vi "Skeleton extraction algorithm (zhangSuen algorithm).vi"() -> ()   [LabVIEW 2021]
panel:
  in  "Input array":dbl[][](array[numeric])=array290x480[139200 elements]
  out "自动迭代次数\nNumber of automatic iterations":i32=4
  in  "automatic 是否自动":bool=TRUE
  out "Step 2":dbl[][](graph)
  in  "指定Zhang-Suen\n     循环次数\nSpecify the number of Zhang-Suen cycles":i32
  out "x与y？":bool
  out "Step 1":dbl[][](graph)
  # "大津算法"
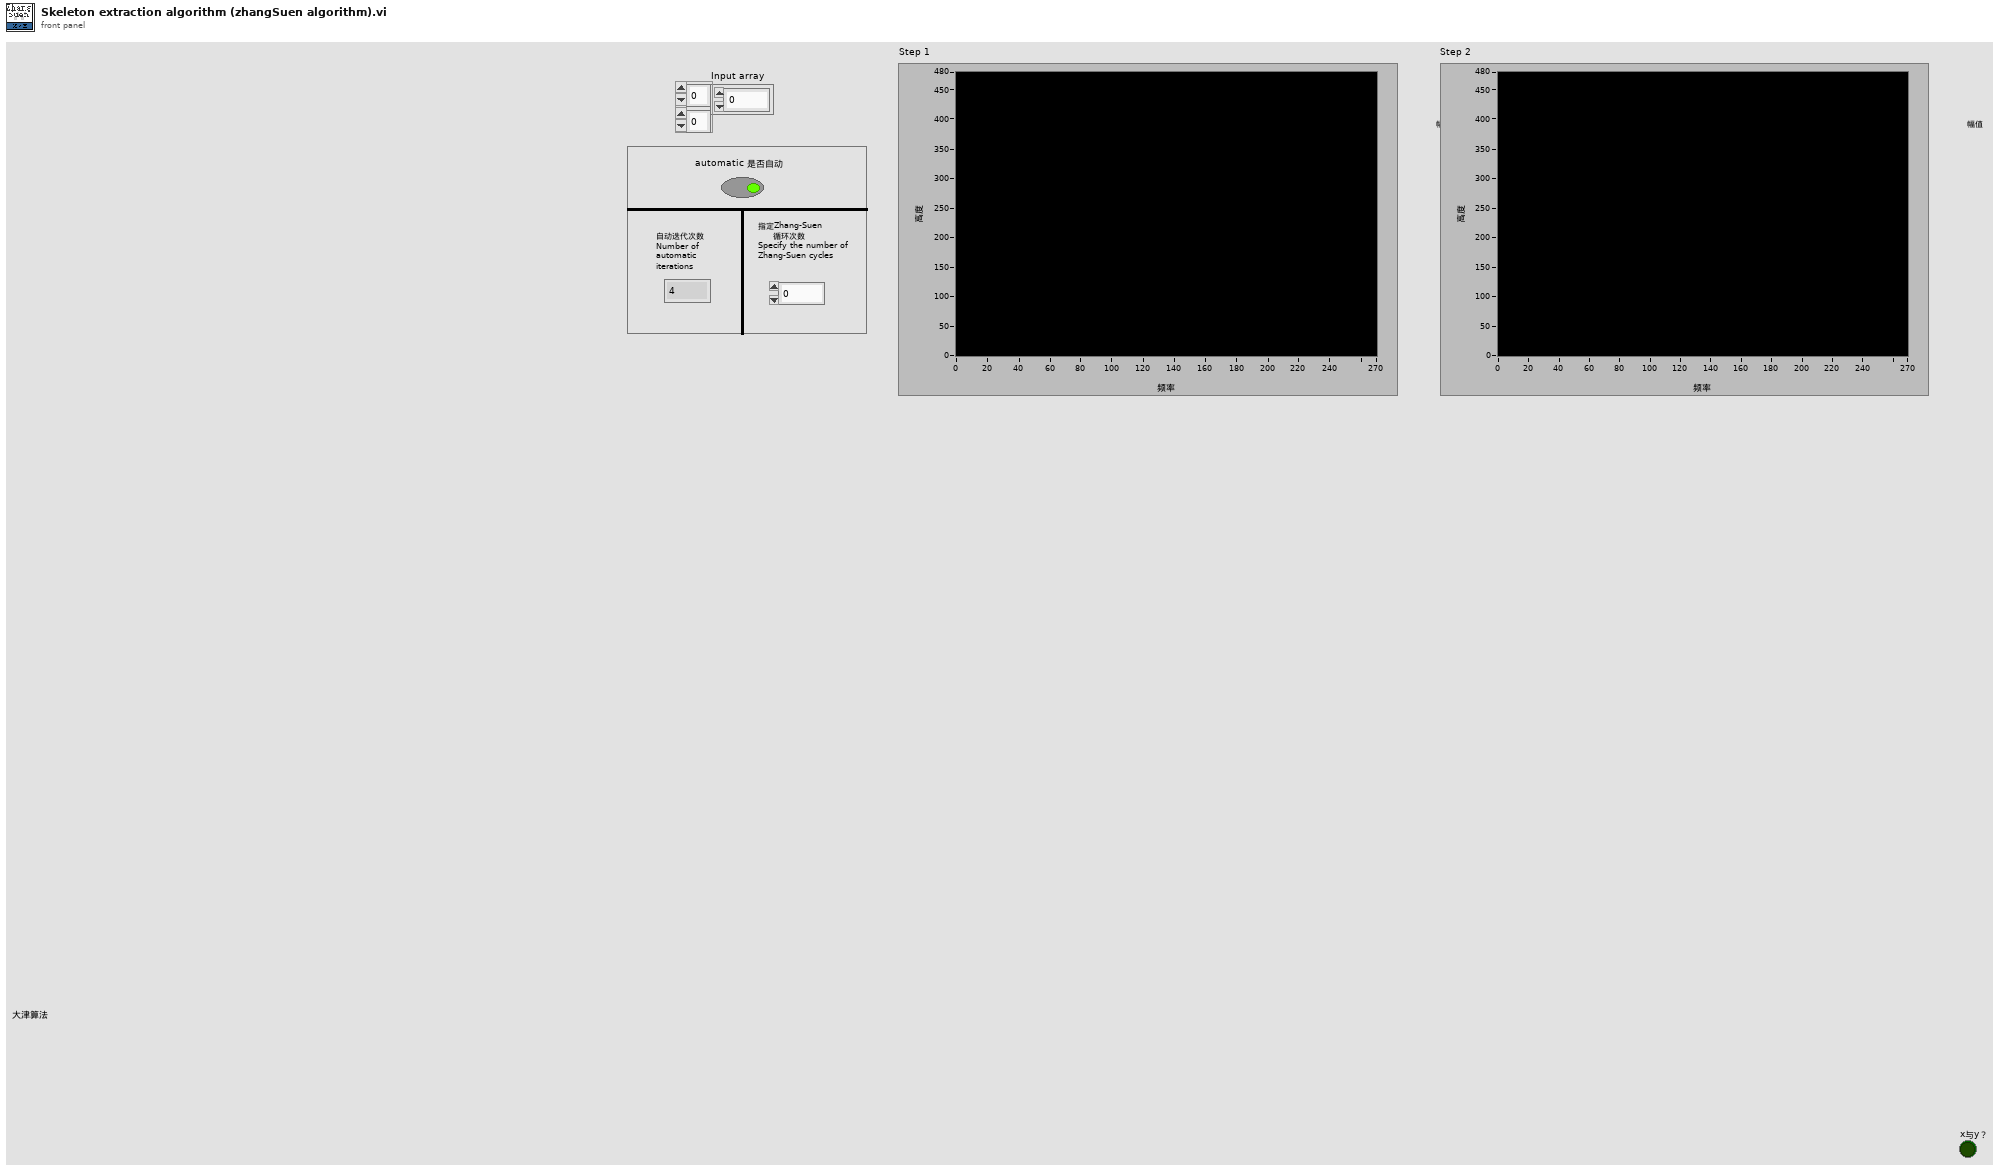
[diagram p1: front panel]
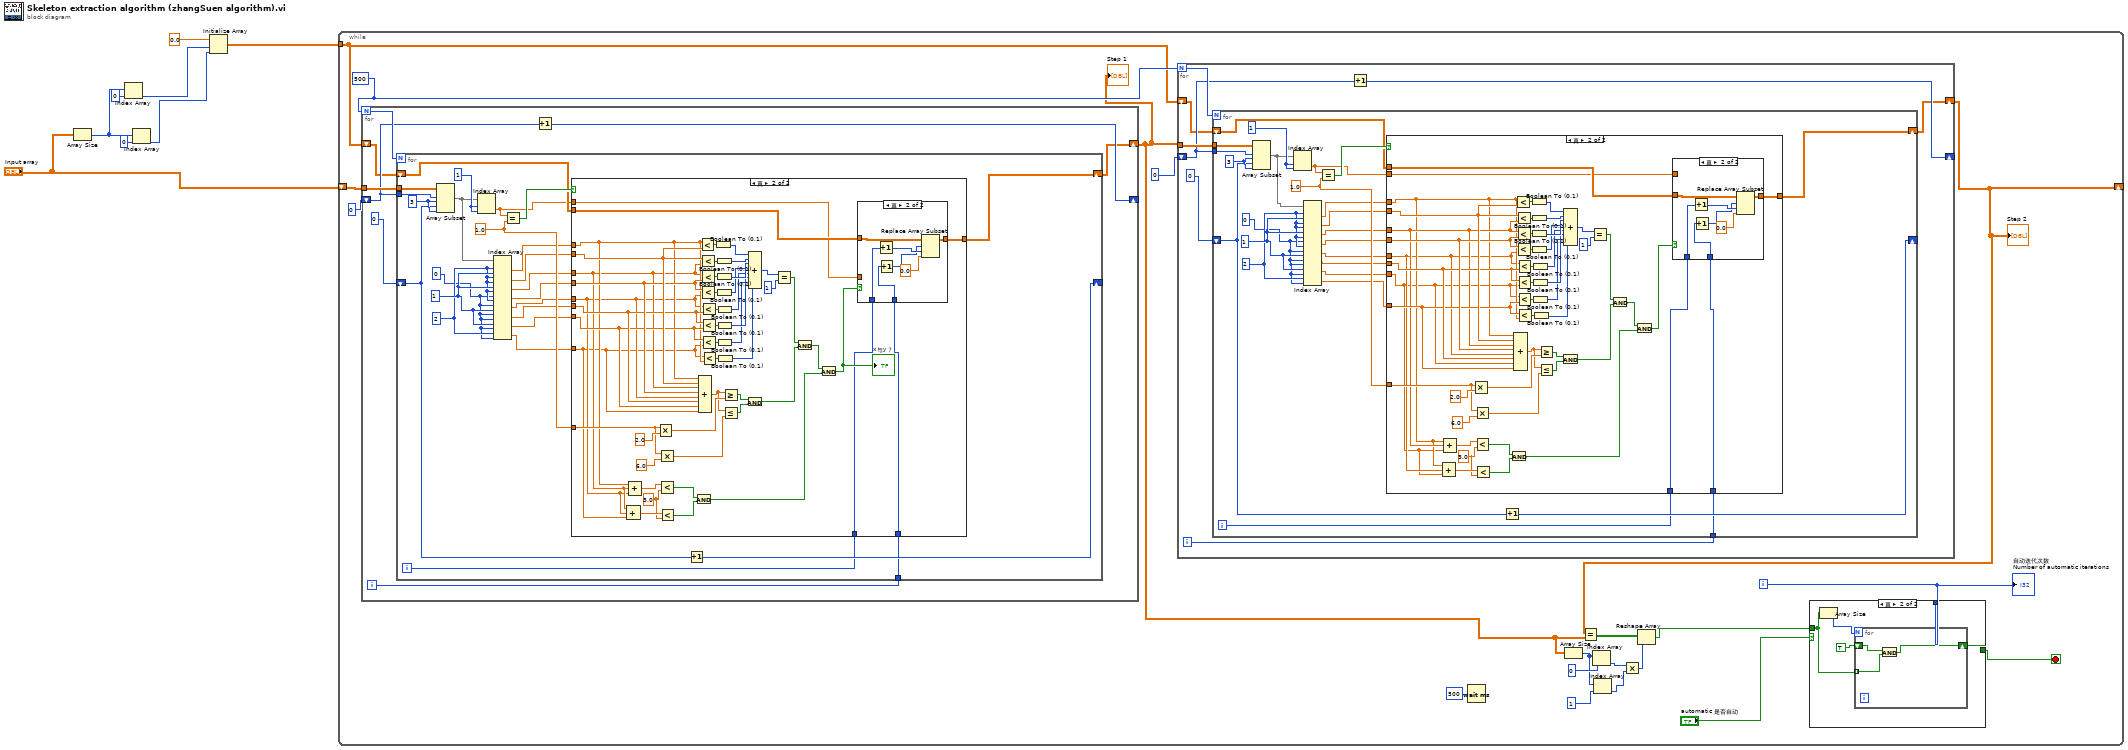
[diagram p0: block diagram]
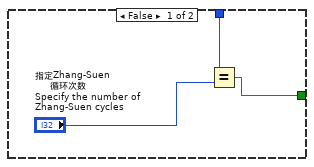
[diagram p2: hidden frame]
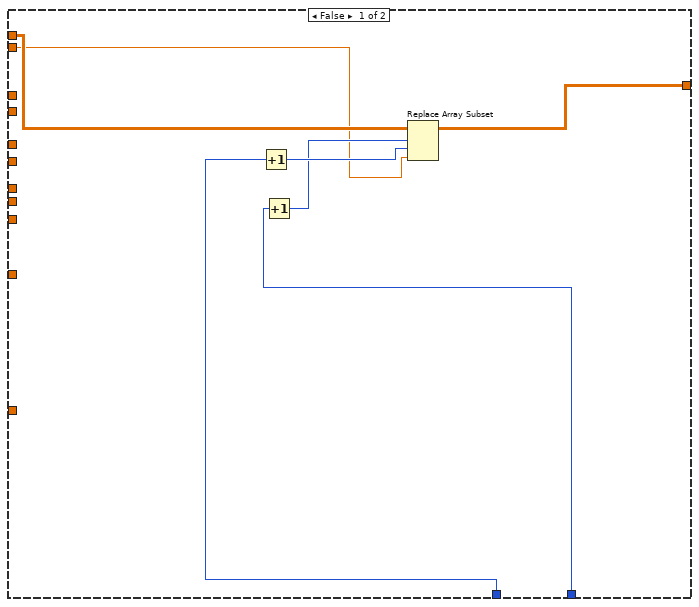
[diagram p3: hidden frame]
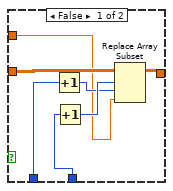
[diagram p4: hidden frame]
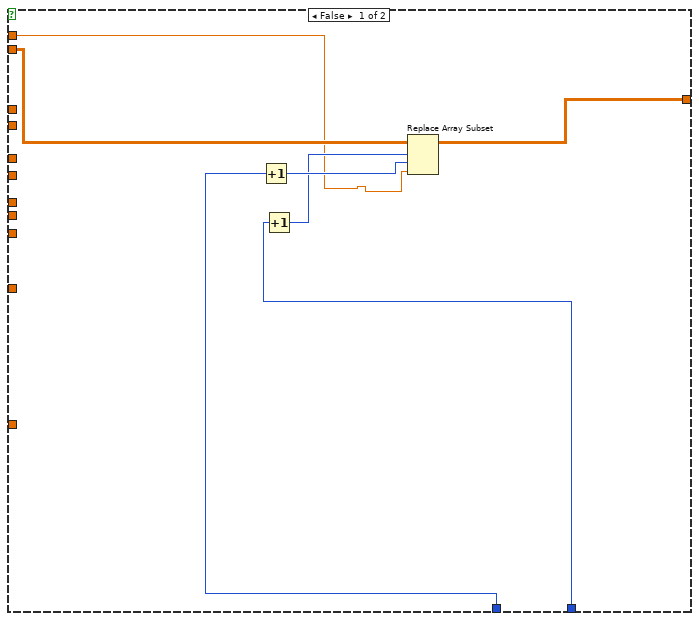
[diagram p5: hidden frame]
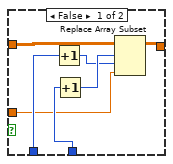
[diagram p6: hidden frame]
diagram:
  n1 = Array Size(array="Input array") -> (size(s)=w2:i32[])
  n2 = Index Array(array=w2, index=0 ("索引")) -> (element=w4:i32)
  n3 = Index Array(array=w2, index=0 ("索引")) -> (element=w1:i32)
  n4 = Initialize Array(0.0 ("元素"), w4, w1) -> (w7:dbl[][])
  n5 = while {
    tunnel: w7 -> [w24]
    shift-right: [w19] -> _
    shift-left: "Input array" -> [w27]
    i -> [w22]
    stop <- w16 stop-if-true
    w25 = 500
    n6 = for {
      N: w25 -> [w147]
      tunnel: w27 -> [w148]
      shift-right: [w145] -> _
      shift-left: 0 ("索引") -> [w146]
      shift-right: [w141] -> w15
      shift-left: w24 -> [w142]
      i -> [w143]
      n7 = for {
        N: w147 -> [_]
        tunnel: w148 -> [w173]
        tunnel: w146 -> [w171]
        shift-right: [w166] -> _
        shift-left: 0 ("索引") -> [w167]
        tunnel: w143 -> [w164]
        shift-right: [w162] -> w141
        shift-left: w142 -> [w163]
        i -> [w165]
        w151 = 2
        w152 = 1
        w150 = 0
        w168 = 1.0 ("新元素/子数组")
        w169 = 1 ("长度")
        w172 = 3 ("长度")
        n8 = Array Subset(array=w173, index (row)=w171, length (row)=w172, index (col)=w167, length (col)=w172) -> (w161:dbl[][])
        n9 = Index Array(array=w161, index (row)=w169, index (col)=w169) -> (element=w149:dbl)
        n10 = Index Array(array=w161, index (row) #1=w151, index (col) #1=w152, index (row) #2=w151, index (col) #2=w151, index (row) #3=w152, index (col) #3=w151, index (row) #4=w150, index (col) #4=w151, index (row) #5=w150, index (col) #5=w152, index (row) #6=w150, index (col) #6=w150, index (row) #7=w152, index (col) #7=w150, index (row) #8=w151, index (col) #8=w150) -> (element #1=w160:dbl, element #2=w159:dbl, element #3=w158:dbl, element #4=w157:dbl, element #5=w156:dbl, element #6=w155:dbl, element #7=w154:dbl, element #8=w153:dbl)
        n11 = Equal?(x=w149, y=w168) -> (x = y?=w170:bool)
        n12 = case shown="真" w170 {
          tunnel: w160 -> [_ w199]
          tunnel: w159 -> [_ w211]
          tunnel: w158 -> [_ w198]
          tunnel: w157 -> [_ w210]
          tunnel: w156 -> [_ w197]
          tunnel: w155 -> [_ w209]
          tunnel: w154 -> [_ w208]
          tunnel: w153 -> [_ w196]
          tunnel: w168 -> [_ w205]
          tunnel: [w180 w185] -> w162
          tunnel: w165 -> [w179 w184]
          tunnel: w164 -> [w176 w183]
          tunnel: w163 -> [w175 w182]
          tunnel: w149 -> [w174 w181]
          frame False {
            n13 = Increment(x=w179) -> (x+1=w178:i32)
            n14 = Increment(x=w176) -> (x+1=w177:i32)
            n15 = Replace Array Subset(array=w175, new element=w174, index (row)=w177, index (col)=w178) -> (w180:dbl[][])
          }
          frame True {
            w193 = 3.0 ("y")
            n16 = Compound Arithmetic op=ADD ("复合运算")(w198, w197, w196) -> (w194:dbl)
            n17 = Compound Arithmetic op=ADD ("复合运算")(w199, w198, w197) -> (w195:dbl)
            n18 = Multiply(x=w205, y=2.0) -> (x*y=w204:dbl)
            n19 = Multiply(x=w205, y=6.0) -> (x*y=w203:dbl)
            n20 = Less?(x=w195, y=w193) -> (x < y?=w192:bool)
            n21 = Less?(x=w194, y=w193) -> (x < y?=w191:bool)
            n22 = And(x=w192, y=w191) -> (x .and. y?=w187:bool)
            n23 = Compound Arithmetic op=ADD ("复合运算")(w199, w211, w198, w210, w197, w209, w208, w196) -> (w202:dbl)
            n24 = Less?(x=w199, y=w211) -> (x < y?=w229:bool)
            n25 = Less?(x=w211, y=w198) -> (x < y?=w228:bool)
            n26 = Less?(x=w198, y=w210) -> (x < y?=w227:bool)
            n27 = Less?(x=w210, y=w197) -> (x < y?=w226:bool)
            n28 = Less?(x=w197, y=w209) -> (x < y?=w225:bool)
            n29 = Less?(x=w209, y=w208) -> (x < y?=w224:bool)
            n30 = Less?(x=w208, y=w196) -> (x < y?=w223:bool)
            n31 = Less?(x=w196, y=w199) -> (x < y?=w222:bool)
            n32 = Boolean To (0,1)(Boolean=w229) -> (0, 1=w221:i16)
            n33 = Boolean To (0,1)(Boolean=w228) -> (0, 1=w220:i16)
            n34 = Boolean To (0,1)(Boolean=w227) -> (0, 1=w219:i16)
            n35 = Boolean To (0,1)(Boolean=w226) -> (0, 1=w218:i16)
            n36 = Boolean To (0,1)(Boolean=w225) -> (0, 1=w217:i16)
            n37 = Boolean To (0,1)(Boolean=w224) -> (0, 1=w216:i16)
            n38 = Boolean To (0,1)(Boolean=w223) -> (0, 1=w215:i16)
            n39 = Boolean To (0,1)(Boolean=w222) -> (0, 1=w214:i16)
            n40 = Greater Or Equal?(x=w202, y=w204) -> (x >= y?=w201:bool)
            n41 = Less Or Equal?(x=w202, y=w203) -> (x <= y?=w200:bool)
            n42 = And(x=w201, y=w200) -> (x .and. y?=w189:bool)
            n43 = Compound Arithmetic op=ADD ("复合运算")(w221, w220, w219, w218, w217, w216, w215, w214) -> (w213:i16)
            n44 = Equal?(x=w213, y=i16 1) -> (x = y?=w190:bool)
            n45 = And(x=w190, y=w189) -> (x .and. y?=w188:bool)
            n46 = And(x=w188, y=w187) -> (x .and. y?=w186:bool)
            "x与y？" <- w186
            n47 = case shown="真" w186 {
              tunnel: w182 -> [w236 w243]
              tunnel: [w235 w241] -> w185
              tunnel: w184 -> [w234 w240]
              tunnel: w183 -> [w233 w239]
              tunnel: w181 -> [w230 _]
              frame False {
                n48 = Increment(x=w234) -> (x+1=w231:i32)
                n49 = Increment(x=w233) -> (x+1=w232:i32)
                n50 = Replace Array Subset(array=w236, new element=w230, index (row)=w232, index (col)=w231) -> (w235:dbl[][])
              }
              frame True {
                n51 = Increment(x=w240) -> (x+1=w238:i32)
                n52 = Increment(x=w239) -> (x+1=w237:i32)
                n53 = Replace Array Subset(array=w243, new element=0.0 ("新元素/子数组"), index (row)=w237, index (col)=w238) -> (w241:dbl[][])
              }
            }
          }
        }
        n54 = Increment(x=w167) -> (x+1=w166:i32)
      }
      n55 = Increment(x=w146) -> (x+1=w145:i32)
    }
    "Step 1" <- w15
    n56 = for {
      N: w25 -> [w44]
      tunnel: w15 -> [w45]
      shift-right: [w42] -> _
      shift-left: 0 ("索引") -> [w43]
      shift-right: [w38] -> w19
      shift-left: w24 -> [w39]
      i -> [w40]
      n57 = for {
        N: w44 -> [_]
        tunnel: w45 -> [w70]
        tunnel: w43 -> [w68]
        shift-right: [w64] -> _
        shift-left: 0 ("索引") -> [w65]
        tunnel: w40 -> [w62]
        shift-right: [w60] -> w38
        shift-left: w39 -> [w61]
        i -> [w63]
        w57 = 2
        w58 = 1
        w56 = 0
        w59 = 1.0 ("新元素/子数组")
        w66 = 1 ("长度")
        w69 = 3 ("长度")
        n58 = Array Subset(array=w70, index (row)=w68, length (row)=w69, index (col)=w65, length (col)=w69) -> (w55:dbl[][])
        n59 = Index Array(array=w55, index (row)=w66, index (col)=w66) -> (element=w46:dbl)
        n60 = Index Array(array=w55, index (row) #1=w57, index (col) #1=w58, index (row) #2=w57, index (col) #2=w57, index (row) #3=w58, index (col) #3=w57, index (row) #4=w56, index (col) #4=w57, index (row) #5=w56, index (col) #5=w58, index (row) #6=w56, index (col) #6=w56, index (row) #7=w58, index (col) #7=w56, index (row) #8=w57, index (col) #8=w56) -> (element #1=w54:dbl, element #2=w53:dbl, element #3=w52:dbl, element #4=w51:dbl, element #5=w50:dbl, element #6=w49:dbl, element #7=w48:dbl, element #8=w47:dbl)
        n61 = Equal?(x=w46, y=w59) -> (x = y?=w67:bool)
        n62 = case shown="真" w67 {
          tunnel: w54 -> [_ w81]
          tunnel: w53 -> [_ w108]
          tunnel: w52 -> [_ w82]
          tunnel: w51 -> [_ w107]
          tunnel: w50 -> [_ w80]
          tunnel: w49 -> [_ w106]
          tunnel: w48 -> [_ w79]
          tunnel: w47 -> [_ w83]
          tunnel: w59 -> [_ w103]
          tunnel: [w77 w87] -> w60
          tunnel: w63 -> [w76 w86]
          tunnel: w62 -> [w73 w85]
          tunnel: w61 -> [w72 w84]
          tunnel: w46 -> [w71 w78]
          frame False {
            n63 = Increment(x=w76) -> (x+1=w75:i32)
            n64 = Increment(x=w73) -> (x+1=w74:i32)
            n65 = Replace Array Subset(array=w72, new element=w71, index (row)=w74, index (col)=w75) -> (w77:dbl[][])
          }
          frame True {
            w95 = 3.0 ("y")
            n66 = Compound Arithmetic op=ADD ("复合运算")(w81, w80, w79) -> (w96:dbl)
            n67 = Compound Arithmetic op=ADD ("复合运算")(w81, w82, w79) -> (w97:dbl)
            n68 = Multiply(x=w103, y=2.0) -> (x*y=w102:dbl)
            n69 = Multiply(x=w103, y=6.0) -> (x*y=w101:dbl)
            n70 = Less?(x=w97, y=w95) -> (x < y?=w94:bool)
            n71 = Less?(x=w96, y=w95) -> (x < y?=w93:bool)
            n72 = And(x=w94, y=w93) -> (x .and. y?=w89:bool)
            n73 = Compound Arithmetic op=ADD ("复合运算")(w81, w108, w82, w107, w80, w106, w79, w83) -> (w100:dbl)
            n74 = Less?(x=w81, y=w108) -> (x < y?=w126:bool)
            n75 = Less?(x=w108, y=w82) -> (x < y?=w125:bool)
            n76 = Less?(x=w82, y=w107) -> (x < y?=w124:bool)
            n77 = Less?(x=w107, y=w80) -> (x < y?=w123:bool)
            n78 = Less?(x=w80, y=w106) -> (x < y?=w122:bool)
            n79 = Less?(x=w106, y=w79) -> (x < y?=w121:bool)
            n80 = Less?(x=w79, y=w83) -> (x < y?=w120:bool)
            n81 = Less?(x=w83, y=w81) -> (x < y?=w119:bool)
            n82 = Boolean To (0,1)(Boolean=w126) -> (0, 1=w118:i16)
            n83 = Boolean To (0,1)(Boolean=w125) -> (0, 1=w117:i16)
            n84 = Boolean To (0,1)(Boolean=w124) -> (0, 1=w116:i16)
            n85 = Boolean To (0,1)(Boolean=w123) -> (0, 1=w115:i16)
            n86 = Boolean To (0,1)(Boolean=w122) -> (0, 1=w114:i16)
            n87 = Boolean To (0,1)(Boolean=w121) -> (0, 1=w113:i16)
            n88 = Boolean To (0,1)(Boolean=w120) -> (0, 1=w112:i16)
            n89 = Boolean To (0,1)(Boolean=w119) -> (0, 1=w111:i16)
            n90 = Greater Or Equal?(x=w100, y=w102) -> (x >= y?=w99:bool)
            n91 = Less Or Equal?(x=w100, y=w101) -> (x <= y?=w98:bool)
            n92 = And(x=w99, y=w98) -> (x .and. y?=w91:bool)
            n93 = Compound Arithmetic op=ADD ("复合运算")(w118, w117, w116, w115, w114, w113, w112, w111) -> (w110:i16)
            n94 = Equal?(x=w110, y=i16 1) -> (x = y?=w92:bool)
            n95 = And(x=w92, y=w91) -> (x .and. y?=w90:bool)
            n96 = And(x=w90, y=w89) -> (x .and. y?=w88:bool)
            n97 = case shown="真" w88 {
              tunnel: w84 -> [w133 w140]
              tunnel: [w132 w138] -> w87
              tunnel: w86 -> [w131 w137]
              tunnel: w85 -> [w130 w136]
              tunnel: w78 -> [w127 _]
              frame False {
                n98 = Increment(x=w131) -> (x+1=w128:i32)
                n99 = Increment(x=w130) -> (x+1=w129:i32)
                n100 = Replace Array Subset(array=w133, new element=w127, index (row)=w129, index (col)=w128) -> (w132:dbl[][])
              }
              frame True {
                n101 = Increment(x=w137) -> (x+1=w135:i32)
                n102 = Increment(x=w136) -> (x+1=w134:i32)
                n103 = Replace Array Subset(array=w140, new element=0.0 ("新元素/子数组"), index (row)=w134, index (col)=w135) -> (w138:dbl[][])
              }
            }
          }
        }
        n104 = Increment(x=w65) -> (x+1=w64:i32)
      }
      n105 = Increment(x=w43) -> (x+1=w42:i32)
    }
    "Step 2" <- w19
    n106 = Wait (ms)(milliseconds to wait=u32 500 ("等待时间（毫秒）")) -> ()  [unwired: 1 out]
    n107 = Array Size(array=w15) -> (size(s)=w12:i32[])
    n108 = Equal?(x=w19, y=w15) -> (x = y?=w18:bool[][])
    n109 = Index Array(array=w12, index=0 ("索引")) -> (element=w11:i32)
    n110 = Index Array(array=w12, index=1 ("索引")) -> (element=w10:i32)
    n111 = Multiply(x=w11, y=w10) -> (x*y=w9:i32)
    n112 = Reshape Array(w18, w9) -> (w17:bool[])
    n113 = case shown="真" "automatic 是否自动" {
      tunnel: [w30 w31] -> w16
      tunnel: w22 -> [w28 _]
      tunnel: w17 -> [_ w32]
      frame False {
        n114 = Equal?(x=w28, y="指定Zhang-Suen\n     循环次数\nSpecify the number of Zhang-Suen cycles") -> (x = y?=w30:bool)
      }
      frame True {
        n115 = Array Size(array=w32) -> (size(s)=w34:i32)
        n116 = for {
          N: w34 -> [_]
          shift-right: [w35] -> w31
          shift-left: TRUE -> [w37]
          tunnel: w32 -> [w36] mode=indexing
          n117 = And(x=w37, y=w36) -> (x .and. y?=w35:bool)
        }
      }
    }
    "自动迭代次数\nNumber of automatic iterations" <- w22
  }
